vi "CloseFifo.vi"(11 "DataLoggingParam":T1={"Fifo Size"=0, "FileRefnum"=refnum, "FifoRefnum"=refnum, "Fifo Time Out (ms)"=500, "MaxNumFileWrite"=255, "Force Num Array"=0}) -> ()   [LabVIEW 2010, in "kevLib2011.lvlib"]
uses:
  kevLib2011.lvlib
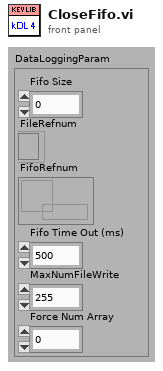
[diagram p1: front panel]
types:
  T1 = cluster{"Fifo Size":u32, "FileRefnum":refnum<file>, "FifoRefnum":refnum<k33>, "Fifo Time Out (ms)":i32, "MaxNumFileWrite":i32, "Force Num Array":i32}
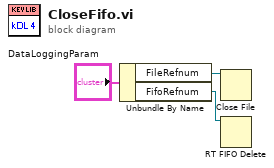
[diagram p0: block diagram]
diagram:
  n1 = Unbundle By Name("DataLoggingParam") -> ("FileRefnum"=w2:refnum<file>, "FifoRefnum"=w1:refnum<k33>)
  n2 = Close File(refnum=w2) -> ()  [unwired: 1 in, 2 out]
  n3 = RT FIFO Delete(0:w1) -> ()  [unwired: 2 in, 1 out]
